vi "Calculate Rake Line Lenghts.vi"(8 "error in (no error)":errorcluster, 10 "Lines Y Distances (non released)":refnum<class "1D Array f32.lvclass">, 11 "Lines X Distances (non released)":refnum<class "1D Array f32.lvclass">) -> (0 "error out":errorcluster, 3 "Rake Line Lengths":refnum<class "1D Array f32.lvclass">)   [LabVIEW 2020, in "G2CPU Line Profile.lvlib"]
uses:
  G2CPU Line Profile.lvlib
  <vilib>/Natan Biesmans/G2CPU GPU and CPU HPC Toolkit/G2CPU Libraries/Arrays/1DArray/f32/1D Array f32.lvclass
  C:/Program Files/National Instruments/LabVIEW 2025/vi.lib/Natan Biesmans/G2CPU GPU and CPU HPC Toolkit/G2CPU Libraries/Arrays/Array/Array Prototype.lvclass
  <vilib>/Natan Biesmans/G2CPU GPU and CPU HPC Toolkit/G2CPU Libraries/Arrays/Array/Array Prototype.lvclass/Array Prototype.ctl
  de018375-398b-436b-8aee-57f370cd140c.vi
  81564c98-21bc-47d8-8253-f7f3c12e33df.vi
  4b1abfa6-574e-4f7b-b58a-022712c137aa.vi
  ff10abd4-7b41-4f35-b37c-ae9ef035f2c1.vi
  <vilib>/Natan Biesmans/G2CPU GPU and CPU HPC Toolkit/G2CPU Libraries/Arrays/Array/G2CPU Get Array Pointer.vi
  de018375-398b-436b-8aee-57f370cd140c.vi/d0fc544b-4239-492d-8a0f-f99369e9c7ae.vi
  de018375-398b-436b-8aee-57f370cd140c.vi/3d9e75e3-2a93-4e4c-a851-83639de319bb.vi
  81564c98-21bc-47d8-8253-f7f3c12e33df.vi/d0fc544b-4239-492d-8a0f-f99369e9c7ae.vi
  81564c98-21bc-47d8-8253-f7f3c12e33df.vi/3d9e75e3-2a93-4e4c-a851-83639de319bb.vi
  4b1abfa6-574e-4f7b-b58a-022712c137aa.vi/5793b77b-c002-4ebf-9075-685617c95341.vi
  4b1abfa6-574e-4f7b-b58a-022712c137aa.vi/2ed3ef86-c00d-4d71-b84c-20267a6dfcf9.vi
  ff10abd4-7b41-4f35-b37c-ae9ef035f2c1.vi/511e4964-6a66-4aff-a71c-0662ce8801c5.vi
  de018375-398b-436b-8aee-57f370cd140c.vi/d0fc544b-4239-492d-8a0f-f99369e9c7ae.vi/6058dca8-195d-4566-b47b-6d6a1c5af61f.vi
  de018375-398b-436b-8aee-57f370cd140c.vi/3d9e75e3-2a93-4e4c-a851-83639de319bb.vi/730f6c57-5c0b-4ee9-b61e-75067b25222b.vi
  de018375-398b-436b-8aee-57f370cd140c.vi/3d9e75e3-2a93-4e4c-a851-83639de319bb.vi/096b8799-7810-404e-baca-ba9279cec4bd.vi
  de018375-398b-436b-8aee-57f370cd140c.vi/3d9e75e3-2a93-4e4c-a851-83639de319bb.vi/0f1a5a47-bcc5-4796-ac31-8dfcfbc0d7d1.vi
  de018375-398b-436b-8aee-57f370cd140c.vi/3d9e75e3-2a93-4e4c-a851-83639de319bb.vi/89f12e17-3330-4b72-ad8f-8dd636660732.vi
  81564c98-21bc-47d8-8253-f7f3c12e33df.vi/d0fc544b-4239-492d-8a0f-f99369e9c7ae.vi/6058dca8-195d-4566-b47b-6d6a1c5af61f.vi
  81564c98-21bc-47d8-8253-f7f3c12e33df.vi/3d9e75e3-2a93-4e4c-a851-83639de319bb.vi/730f6c57-5c0b-4ee9-b61e-75067b25222b.vi
  81564c98-21bc-47d8-8253-f7f3c12e33df.vi/3d9e75e3-2a93-4e4c-a851-83639de319bb.vi/096b8799-7810-404e-baca-ba9279cec4bd.vi
  81564c98-21bc-47d8-8253-f7f3c12e33df.vi/3d9e75e3-2a93-4e4c-a851-83639de319bb.vi/0f1a5a47-bcc5-4796-ac31-8dfcfbc0d7d1.vi
  81564c98-21bc-47d8-8253-f7f3c12e33df.vi/3d9e75e3-2a93-4e4c-a851-83639de319bb.vi/89f12e17-3330-4b72-ad8f-8dd636660732.vi
  4b1abfa6-574e-4f7b-b58a-022712c137aa.vi/5793b77b-c002-4ebf-9075-685617c95341.vi/3e802c67-fb96-46a3-ae13-4994a8508b4f.vi
  4b1abfa6-574e-4f7b-b58a-022712c137aa.vi/5793b77b-c002-4ebf-9075-685617c95341.vi/5a50fc67-79e7-4972-80c2-92243cd53dd4.vi
  4b1abfa6-574e-4f7b-b58a-022712c137aa.vi/2ed3ef86-c00d-4d71-b84c-20267a6dfcf9.vi/730f6c57-5c0b-4ee9-b61e-75067b25222b.vi
  4b1abfa6-574e-4f7b-b58a-022712c137aa.vi/2ed3ef86-c00d-4d71-b84c-20267a6dfcf9.vi/096b8799-7810-404e-baca-ba9279cec4bd.vi
  4b1abfa6-574e-4f7b-b58a-022712c137aa.vi/2ed3ef86-c00d-4d71-b84c-20267a6dfcf9.vi/0f1a5a47-bcc5-4796-ac31-8dfcfbc0d7d1.vi
  4b1abfa6-574e-4f7b-b58a-022712c137aa.vi/2ed3ef86-c00d-4d71-b84c-20267a6dfcf9.vi/89f12e17-3330-4b72-ad8f-8dd636660732.vi
  de018375-398b-436b-8aee-57f370cd140c.vi/d0fc544b-4239-492d-8a0f-f99369e9c7ae.vi/6058dca8-195d-4566-b47b-6d6a1c5af61f.vi/77c7badc-ed81-4514-99c1-20d37f4e5ecc.vi
  de018375-398b-436b-8aee-57f370cd140c.vi/d0fc544b-4239-492d-8a0f-f99369e9c7ae.vi/6058dca8-195d-4566-b47b-6d6a1c5af61f.vi/eb76fa01-6782-47b4-b34f-9eb474c9cc78.vi
  <vilib>/Natan Biesmans/G2CPU GPU and CPU HPC Toolkit/ArrayFire Driver/VIs/Run as Multi Device.vi
  81564c98-21bc-47d8-8253-f7f3c12e33df.vi/d0fc544b-4239-492d-8a0f-f99369e9c7ae.vi/6058dca8-195d-4566-b47b-6d6a1c5af61f.vi/77c7badc-ed81-4514-99c1-20d37f4e5ecc.vi
  81564c98-21bc-47d8-8253-f7f3c12e33df.vi/d0fc544b-4239-492d-8a0f-f99369e9c7ae.vi/6058dca8-195d-4566-b47b-6d6a1c5af61f.vi/eb76fa01-6782-47b4-b34f-9eb474c9cc78.vi
  <vilib>/Natan Biesmans/G2CPU GPU and CPU HPC Toolkit/ArrayFire Driver/VIs/iszero.vi
  <vilib>/Natan Biesmans/G2CPU GPU and CPU HPC Toolkit/ArrayFire Driver/VIs/sub.vi
  <vilib>/Natan Biesmans/G2CPU GPU and CPU HPC Toolkit/ArrayFire Driver/VIs/release array.vi
  <vilib>/Natan Biesmans/G2CPU GPU and CPU HPC Toolkit/ArrayFire Driver/subvi/Error Converter (ErrCode or Status).vi
  <vilib>/Natan Biesmans/G2CPU GPU and CPU HPC Toolkit/ArrayFire Driver/VIs/cast.vi
  <vilib>/Natan Biesmans/G2CPU GPU and CPU HPC Toolkit/ArrayFire Driver/VIs/add.vi
  <vilib>/Natan Biesmans/G2CPU GPU and CPU HPC Toolkit/G2CPU Libraries/Arrays/Array/G2CPU Set Array Pointer.vi
  <vilib>/Natan Biesmans/G2CPU GPU and CPU HPC Toolkit/G2CPU Libraries/Arrays/SubVI/is 1D.vi
  <vilib>/Natan Biesmans/G2CPU GPU and CPU HPC Toolkit/ArrayFire Driver/VIs/pow.vi
  <vilib>/Natan Biesmans/G2CPU GPU and CPU HPC Toolkit/G2CPU Libraries/Arrays/Array/G2CPU Release Array.vi
  <vilib>/Natan Biesmans/G2CPU GPU and CPU HPC Toolkit/ArrayFire Driver/VIs/sqrt.vi
  <vilib>/Natan Biesmans/G2CPU GPU and CPU HPC Toolkit/G2CPU Libraries/Arrays/Array/Array Prototype.lvclass
  <vilib>/Natan Biesmans/G2CPU GPU and CPU HPC Toolkit/G2CPU Libraries/Arrays/1DArray/1D Array Prototype.lvclass
  <vilib>/Natan Biesmans/G2CPU GPU and CPU HPC Toolkit/G2CPU Libraries/Arrays/DataTypes/f32/f32.lvclass
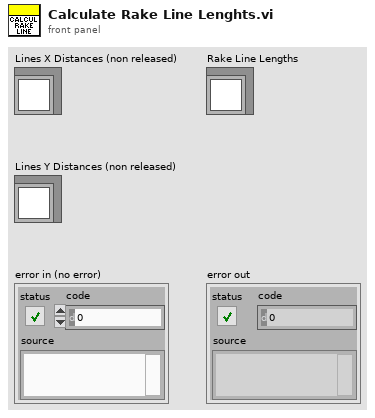
[diagram p1: front panel]
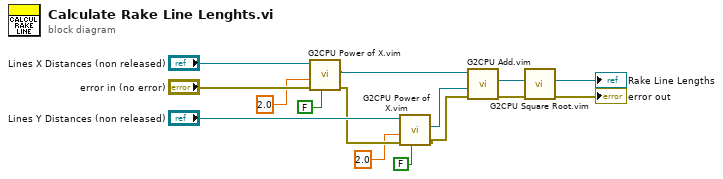
[diagram p0: block diagram]
diagram:
  n1 = call "G2CPU Power of X.vim"("Auto Release lhs (Enabled)"=FALSE, "error in (no error)"="error in (no error)", "Array rhs"=sgl 2.0 ("Datatype"), "Array lhs"="Lines X Distances (non released)") -> ("error out"=w14:errorcluster, "Array Result"=w6:refnum<class "1D Array f32.lvclass">)  [unwired: 6 in]
  n2 = call "G2CPU Power of X.vim"("Auto Release lhs (Enabled)"=FALSE, "error in (no error)"=w14, "Array rhs"=sgl 2.0 ("Datatype"), "Array lhs"="Lines Y Distances (non released)") -> ("error out"=w12:errorcluster, "Array Result"=w13:refnum<class "1D Array f32.lvclass">)  [unwired: 6 in]
  n3 = call "G2CPU Add.vim"("error in (no error)"=w12, "Array rhs"=w13, "Array lhs"=w6) -> ("error out"=w4:errorcluster, "Array Result"=w1:refnum<class "1D Array f32.lvclass">)  [unwired: 7 in]
  n4 = call "G2CPU Square Root.vim"("error in (no error)"=w4, "Array in"=w1) -> ("error out"=→"error out":errorcluster, "Array Result"=→"Rake Line Lengths":refnum<class "1D Array f32.lvclass">)  [unwired: 8 in]
